vi "LastConfig.vi"(8 "errin":errorcluster, 11 "Application Directory":path) -> (0 "error out":errorcluster, 3 "Derniere Config":string)   [LabVIEW 2020]
panel:
  out "element":string
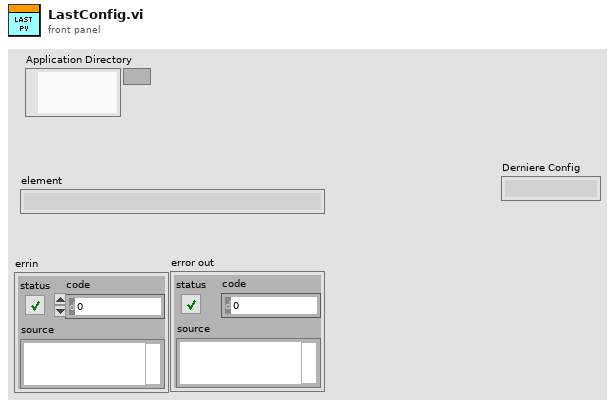
[diagram p1: front panel]
types:
  T1 = cluster{"Status":string, "SN":string, "Date test":string, "SOC":string, "Config":string}
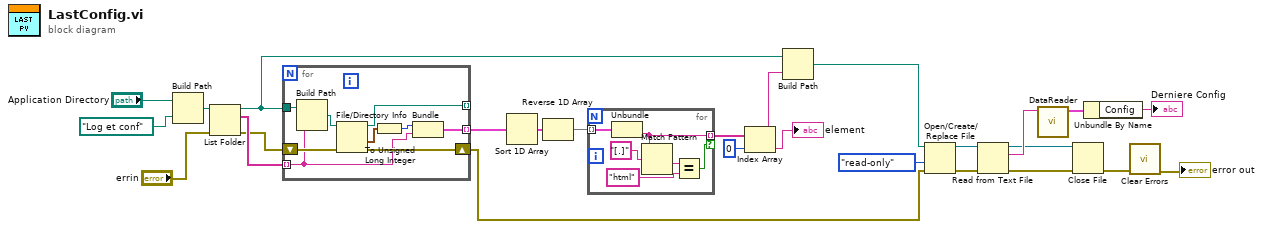
[diagram p0: block diagram]
diagram:
  n1 = Build Path(base path="Application Directory", name or relative path=path "Log et conf") -> (appended path=w18:path)
  n2 = List Folder(path=w18, error in="errin") -> (path out=w12:path, filenames=w23:string[], error out=w22:errorcluster)  [unwired: 2 in, 1 out]
  n3 = for {
    tunnel: w12 -> [w32]
    tunnel: w23 -> [w29] mode=indexing
    shift-right: [w30] -> w9
    shift-left: w22 -> [w31]
    tunnel: [w28] -> w24 mode=indexing
    tunnel: [w26] -> _ mode=indexing
    n4 = Build Path(base path=w32, name or relative path=w29) -> (appended path=w27:path)
    n5 = File/Directory Info(path=w27, error in=w31) -> (path out=w26:path, last mod=w33:timestamp, error out=w30:errorcluster)  [unwired: 4 out]
    n6 = To Unsigned Long Integer(number=w33) -> (unsigned 32bit integer=w34:u32)
    n7 = Bundle(w34, w29) -> (w28:cluster{u32, string})  [unwired: 1 in]
  }
  n8 = Sort 1D Array(array=w24) -> (sorted array=w25:cluster{u32, string}[])
  n9 = Reverse 1D Array(array=w25) -> (reversed array=w17:cluster{u32, string}[])
  n10 = for {
    tunnel: w17 -> [w40] mode=indexing
    tunnel: [w38] -> w16 mode=indexing if=w35
    n11 = Unbundle(w40) -> (w38:string)  [unwired: 1 out]
    n12 = Match Pattern(string=w38, regular expression="[.]") -> (after substring=w37:string)  [unwired: 1 in, 3 out]
    n13 = Equal?(x=w37, y="html") -> (x = y?=w35:bool)
  }
  n14 = Index Array(array=w16, index=0) -> (element=w11:string)
  "element" <- w11
  n15 = Build Path(base path=w12, name or relative path=w11) -> (appended path=w10:path)
  n16 = Open/Create/Replace File(file path (use dialog)=w10, error in=w9, access (0:read/write)=enum16{"read/write", "read-only", "write-only"}."read-only") -> (refnum out=w13:refnum<file>, error out=w14:errorcluster)  [unwired: 3 in, 1 out]
  n17 = Read from Text File(file (use dialog)=w13, error in=w14) -> (refnum out=w5:refnum<file>, text=w7:string, error out=w6:errorcluster)  [unwired: 2 in, 1 out]
  n18 = call "DataReader.vi"("PV html"=w7) -> ("Cluster"=w4:T1)  [unwired: 10 in]
  n19 = Close File(refnum=w5, error in=w6) -> (error out=w2:errorcluster)  [unwired: 1 out]
  n20 = Unbundle By Name(w4) -> ("Config"=→"Derniere Config":string)
  n21 = call <vilib>:"Clear Errors.vi"("error in (no error)"=w2) -> ("error out"=→"error out":errorcluster)  [unwired: 5 in, 1 out]
